vi "Read Register.vi"(0 "Refnum in":refnum<visa-resource-name>, 1 "startReg":u16, 2 "Quantity":u16=1, 5 "Mode":T1, 9 "Register type":enum16{"Input", "Holding"}(ring), 11 "error in (no error)":errorcluster, 12 "Enable":bool) -> (4 "Refnum Out":refnum<visa-resource-name>, 6 "ModeOut":T1, 8 "Holding Registers":u16[](array[numeric]), 10 "Numeric":u16, 15 "error out":errorcluster)   [LabVIEW 2020]
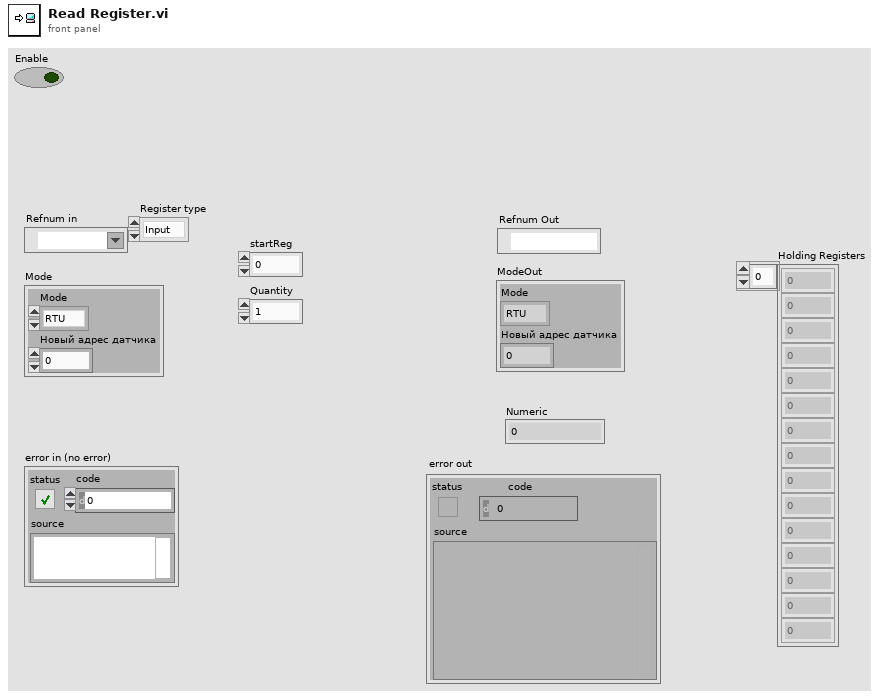
[diagram p1: front panel]
types:
  T1 = cluster{"Mode":enum16{"RTU", "ASCII"}, "Новый адрес датчика":u16}
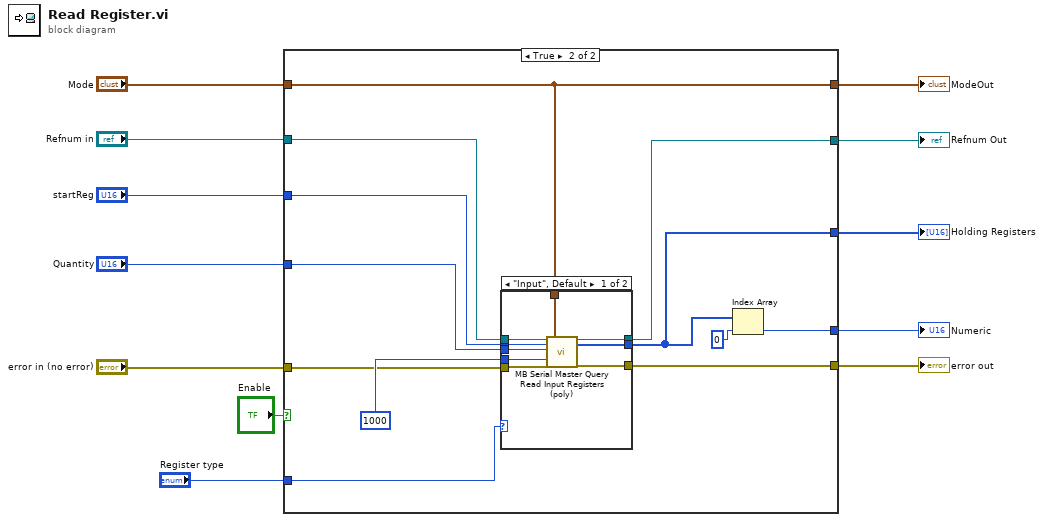
[diagram p0: block diagram]
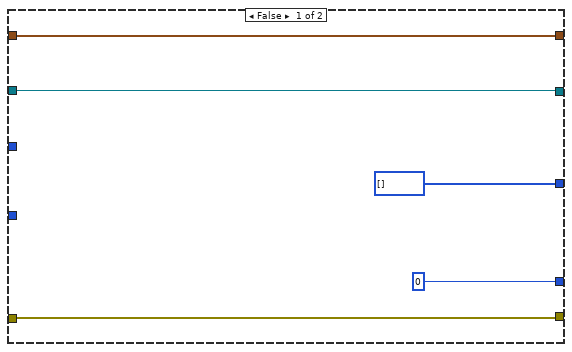
[diagram p2: hidden frame]
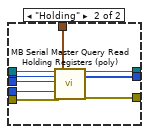
[diagram p3: hidden frame]
diagram:
  n1 = case shown="True" "Enable" {
    tunnel: [u16[] [] ("Holding Registers") w19] -> w12
    tunnel: "Mode" -> [w16 w23]
    tunnel: "error in (no error)" -> [w17 w27]
    tunnel: "Refnum in" -> [w15 w22]
    tunnel: "startReg" -> [_ w26]
    tunnel: "Quantity" -> [_ w20]
    tunnel: [u16 0 ("Numeric") w25] -> w7
    tunnel: [w17 w24] -> w6
    tunnel: [w16 w23] -> w4
    tunnel: [w15 w21] -> w3
    tunnel: "Register type" -> [_ w18]
    frame False {
    }
    frame True {
      n2 = case shown="\"Input\", Default" w18 {
        tunnel: u32 1000 ("Timeout") -> [w32 w47]
        tunnel: w27 -> [w31 w46]
        tunnel: w26 -> [w35 w45]
        tunnel: [w30 w44] -> w24
        tunnel: w23 -> [w38 w43]
        tunnel: w22 -> [w37 w42]
        tunnel: [w36 w41] -> w21
        tunnel: w20 -> [w34 w40]
        tunnel: [w33 w39] -> w19
        frame "Input", Default {
          n3 = call <vilib>:"MB Serial Master Query Read Input Registers (poly).vi"("VISA resource name"=w37, "Starting Address"=w35, "Quantity"=w34, "Timeout"=w32, "error in"=w31, "Serial Parameters"=w38) -> ("VISA resource name out"=w36:refnum<visa-resource-name>, "Input Registers"=w33:u16[], "error out"=w30:errorcluster)  [unwired: 10 in, 1 out]
        }
        frame "Holding" {
          n4 = call <vilib>:"MB Serial Master Query Read Holding Registers (poly).vi"("VISA resource name"=w42, "Starting Address"=w45, "Quantity"=w40, "Timeout"=w47, "error in"=w46, "Serial Parameters"=w43) -> ("VISA resource name out"=w41:refnum<visa-resource-name>, "Holding Registers"=w39:u16[], "error out"=w44:errorcluster)  [unwired: 10 in, 1 out]
        }
      }
      n5 = Index Array(array=w19, index=u16 0 ("Starting Address")) -> (element=w25:u16)
    }
  }
  "Numeric" <- w7
  "error out" <- w6
  "ModeOut" <- w4
  "Refnum Out" <- w3
  "Holding Registers" <- w12
